vi "Read String Range.vi"(0 "Report Ref In":T1, 1 "Row Count":i32=1, 2 "Start Row Index":i32, 3 "Start Column Index":i32, 4 "Column Count":i32=1, 5 "error in (no error)":errorcluster) -> (6 "Report Ref Out":T1, 7 "Output Range":string[][](array[string]), 8 "error out":errorcluster)   [LabVIEW 2026, in "XCel Report Engine.lvlib"]
uses:
  XCel Report Engine.lvlib
  Controls/Report Ref.ctl
  C:/Users/m.santucci/Documents/ChatGPT/LV_REPORT_ENGINE/.net/src/XCelReportEngine/bin/Release/net48/XCelReportEngine.dll
  .net/src/XCelReportEngine/bin/Release/net48/XCelReportEngine.dll
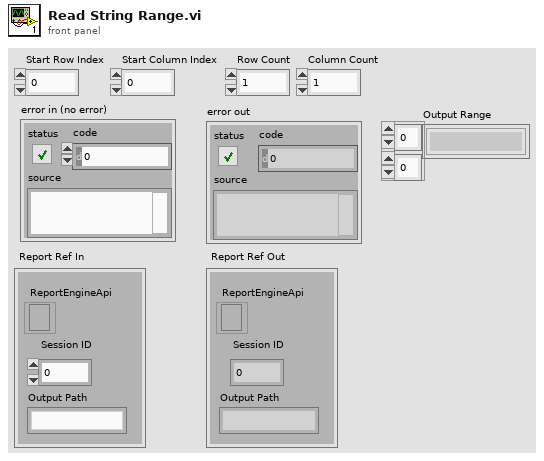
[diagram p1: front panel]
types:
  T1 = typedef "XCel Report Engine.lvlib/Report Ref.ctl" = cluster{"Session ID":i32, "Output Path":string, "ReportEngineApi":refnum<k24>}
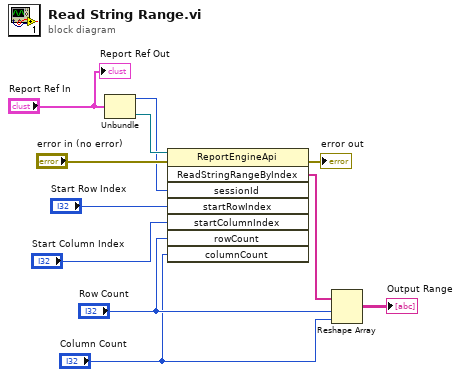
[diagram p0: block diagram]
diagram:
  n1 = Unbundle("Report Ref In") -> ("Session ID"=w7:i32, "ReportEngineApi"=w10:refnum<k24>)  [unwired: 1 out]
  n2 = invoke class="ReportEngineApi" method="ReadStringRangeByIndex"(reference=w10, error in="error in (no error)", "sessionId"=w7, "startRowIndex"="Start Row Index", "startColumnIndex"="Start Column Index", "rowCount"="Row Count", "columnCount"="Column Count") -> (error out=→"error out":errorcluster, "ReadStringRangeByIndex"=w4:string[])  [unwired: 1 in, 6 out]
  n3 = Reshape Array(w4, "Row Count", "Column Count") -> (→"Output Range":string[][])
  "Report Ref Out" <- "Report Ref In"
